vi "NF87XX.relative move.vi"(0 "i ref in":refnum<vi>, 1 "steps (-2147483648 .. 2147483648)":i32, 2 "acceleration (16 .. 20000)":dbl=16.0 min=16.0 max=20000.0, 3 "start velocity (0 .. 1999)":dbl min=0.0 max=1999.0, 4 "velocity (1 .. 2000)":dbl=1.0 min=1.0 max=2000.0, 5 "error in (no error)":errorcluster, 6 "Motor (0, 1 or 2)":i32, 7 "System":string) -> (14 "i ref out":refnum<vi>, 19 "error out":errorcluster)   [LabVIEW 2014, in "NF87XX.lvlib"]
doc: "This VI sets acceleration, start velocity and velocity. Depending on the sign, it moves the specified axis forward or back by the number of steps given. The value for the axis should be within 0..2. This case is forseen for 3-channel open loop drivers only.\n\nauthor: Stefan Götte\ndata: 09-JAN-2007\n\nLicense Agreement for this software:\n\nCopyright (C)\nGesellschaft für Schwerionenforschung, GSI\nPlanckstr. 1\n64291 Darmstadt\nGermany\n\nContact: D.Beck@gsi.de \n\nThis program is free software; you can redistribute it and/or modify it under the terms of the GNU General Public License as published by the Free Software Foundation; either version 2 of the license, or (at your option) any later version.\n\nThis program is distributed in the hope that it will be useful, but WITHOUT ANY WARRANTY; without even the implied warranty of MERCHANTABILITY or FITNESS FOR A PARTICULAR PURPOSE. See the GNU General License for more details (http://www.gnu.org).\n\nGesellschaft für Schwerionenforschung, GSI\nPlanckstr. 1, 64291 Darmstadt, Germany\nFor all questions and ideas contact: M.Richter@gsi.de, H.Brand@gsi.de or D.Beck@gsi.de.\nLast update: 17-JUN-2004"
uses:
  NF87XX.lvlib
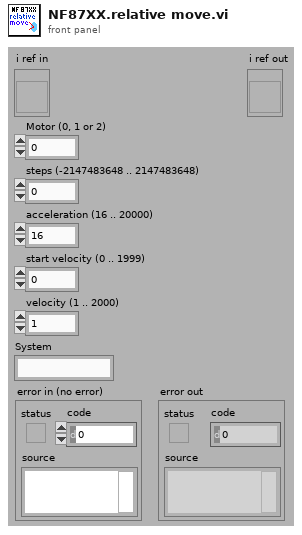
[diagram p1: front panel]
types:
  T1 = typedef "NF87XX.lvlib/NF87XX.driver Type.ctl" = enum16{"not defined", "3-ch open loop drv", "1-ch closed loop drv"}
  T2 = typedef "NF87XX.lvlib/NF87XX.i attribute.ctl" = cluster{"Con Settings":T3, "Drivers":T4[], "Status":cluster{"Service ID":i32, "Status":T6}, "Joystick available":bool, "VISA Resource":string}
  T3 = typedef "NewFocusPico - Driver np.lvlib/VISA & TCPIP Control.ctl" = cluster{"VISA or TCP/IP":bool, "Init Connection":bool, "Close Connection":bool, "Resource Name":refnum<visa-resource-name>, "hostname":string, "connection ID":refnum<k5>}
  T4 = typedef "NF87XX.lvlib/NF87XX.driver Settings.ctl" = cluster{"Name":string, "Driver Type":T1, "Pico Parameter type":T5, "Acceleration [Steps/s²]":cluster{"Motor 0":dbl, "Motor 1":dbl, "Motor 2":dbl}, "Start Velocity [Steps/s]":cluster{"Motor 0":dbl, "Motor 1":dbl, "Motor 2":dbl}, "Velocity [Steps/s]":cluster{"Motor 0":dbl, "Motor 1":dbl, "Motor 2":dbl}, "axis channel":i32, "Position":i32, "Position Service ID":i32}
  T5 = typedef "NewFocusPico - Driver np.lvlib/Pico Parameters.ctl" = cluster{"Pico Type":enum16{"Open-Loop Pico", "Close-Loop Pico", "Pico Ultra"}, "Acceleration (steps/sec^2)":string, "Velocity ( Hz)":string, "Driver":string, "Motor":string, "Channel":string, "Process Step":string}
  T6 = typedef "PH_StatusHandler.lvlib/PH_StatusHandler.Status.ctl" = i16
  T7 = cluster{"Motor 0":dbl, "Motor 1":dbl, "Motor 2":dbl}
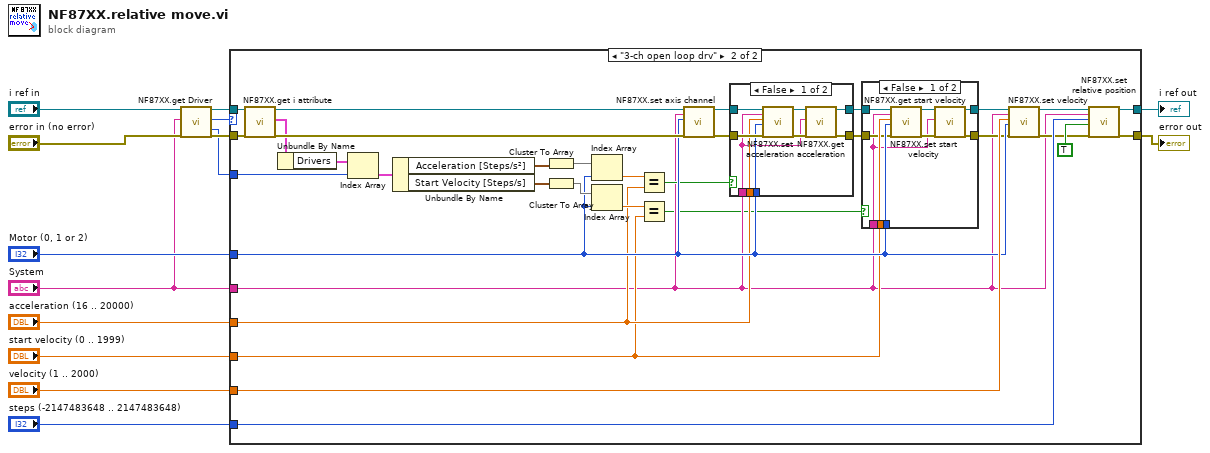
[diagram p0: block diagram]
diagram:
  n1 = call "NF87XX.get Driver.vi"("i ref in"="i ref in", "System"="System", "error in (no error)"="error in (no error)") -> ("i ref out"=w4:refnum<vi>, "Driver Type"=w2:T1, "Driver Index"=w1:i32, "error out"=w6:errorcluster)  [unwired: 12 in, 1 out]
  n2 = case shown="\"3-ch open loop drv\"" w2 {
    tunnel: "steps (-2147483648 .. 2147483648)" -> [_ w49]
    tunnel: "Motor (0, 1 or 2)" -> [_ w28]
    tunnel: "acceleration (16 .. 20000)" -> [_ w25]
    tunnel: "start velocity (0 .. 1999)" -> [_ w24]
    tunnel: "velocity (1 .. 2000)" -> [_ w43]
    tunnel: [w16 w42] -> w9
    tunnel: [w15 w41] -> w8
    tunnel: w6 -> [w15 w38]
    tunnel: w4 -> [w16 w40]
    tunnel: "System" -> [_ w18]
    tunnel: w1 -> [_ w34]
    frame "not defined", Default {
    }
    frame "3-ch open loop drv" {
      n3 = call "NF87XX.get i attribute.vi"("i ref in"=w40, "error in (no error)"=w38) -> ("i ref out"=w39:refnum<vi>, "i attribute"=w36:T2, "error out"=w37:errorcluster)  [unwired: 15 in]
      n4 = Unbundle By Name(w36) -> ("Drivers"=w35:T4[])
      n5 = Index Array(array=w35, index=w34) -> (element=w33:T4)
      n6 = Unbundle By Name(w33) -> ("Acceleration [Steps/s²]"=w32:T7, "Start Velocity [Steps/s]"=w31:T7)
      n7 = Cluster To Array(cluster=w32) -> (array=w30:dbl[])
      n8 = Cluster To Array(cluster=w31) -> (array=w29:dbl[])
      n9 = Index Array(array=w30, index=w28) -> (element=w27:dbl)
      n10 = Index Array(array=w29, index=w28) -> (element=w26:dbl)
      n11 = Equal?(x=w27, y=w25) -> (x = y?=w21:bool)
      n12 = Equal?(x=w26, y=w24) -> (x = y?=w17:bool)
      n13 = call "NF87XX.set axis channel.vi"("i ref in"=w39, "System"=w18, "channel"=w28, "error in (no error)"=w37) -> ("i ref out"=w45:refnum<vi>, "error out"=w47:errorcluster)  [unwired: 14 in]
      n14 = case shown="False" w21 {
        tunnel: w47 -> [w69 w70]
        tunnel: w45 -> [w68 w71]
        tunnel: w28 -> [w67 _]
        tunnel: w25 -> [w66 _]
        tunnel: [w64 w71] -> w23
        tunnel: [w62 w70] -> w22
        tunnel: w18 -> [w61 _]
        frame False {
          n15 = call "NF87XX.set acceleration.vi"("i ref in"=w68, "System"=w61, "acceleration (16 .. 20000)"=w66, "Motor (0,1,2)"=w67, "error in (no error)"=w69) -> ("i ref out"=w65:refnum<vi>, "error out"=w63:errorcluster)  [unwired: 13 in]
          n16 = call "NF87XX.get acceleration.vi"("i ref in"=w65, "System"=w61, "error in (no error)"=w63) -> ("i ref out"=w64:refnum<vi>, "error out"=w62:errorcluster)  [unwired: 12 in, 3 out]
        }
        frame True {
        }
      }
      n17 = case shown="False" w17 {
        tunnel: w28 -> [w58 _]
        tunnel: w24 -> [w57 _]
        tunnel: w23 -> [w56 w60]
        tunnel: w22 -> [w55 w59]
        tunnel: [w53 w60] -> w20
        tunnel: [w51 w59] -> w19
        tunnel: w18 -> [w50 _]
        frame False {
          n18 = call "NF87XX.set start velocity.vi"("i ref in"=w56, "System"=w50, "start velocity (0 .. 1999)"=w57, "Motor (0,1,2)"=w58, "error in (no error)"=w55) -> ("i ref out"=w54:refnum<vi>, "error out"=w52:errorcluster)  [unwired: 13 in]
          n19 = call "NF87XX.get start velocity.vi"("i ref in"=w54, "System"=w50, "error in (no error)"=w52) -> ("i ref out"=w53:refnum<vi>, "error out"=w51:errorcluster)  [unwired: 12 in, 3 out]
        }
        frame True {
        }
      }
      n20 = call "NF87XX.set velocity.vi"("i ref in"=w20, "System"=w18, "velocity (1 .. 2000)"=w43, "Motor (0,1,2)"=w28, "error in (no error)"=w19) -> ("i ref out"=w44:refnum<vi>, "error out"=w46:errorcluster)  [unwired: 13 in]
      n21 = call "NF87XX.set relative position.vi"("i ref in"=w44, "System"=w18, "steps"=w49, "Go immediately?"=TRUE, "error in (no error)"=w46) -> ("i ref out"=w42:refnum<vi>, "error out"=w41:errorcluster)  [unwired: 13 in]
    }
  }
  "error out" <- w8
  "i ref out" <- w9
